vi "PainfulTrial.vi"() -> ()   [LabVIEW 2016]
uses:
  <vilib>/express/express arith-compare/Formula/XNode/ExpressFormulaBlockNode.xnode
panel:
  out "d (m) 2":dbl
  in  "D (in) 2":dbl
  in  "E (psi) 2":dbl
  in  "L (in) 2":dbl
  in  "F (Lbf) 2":dbl
  out "d (m)":dbl
  in  "D (in)":dbl
  in  "E (psi)":dbl
  in  "L (in)":dbl
  in  "F (Lbf)":dbl
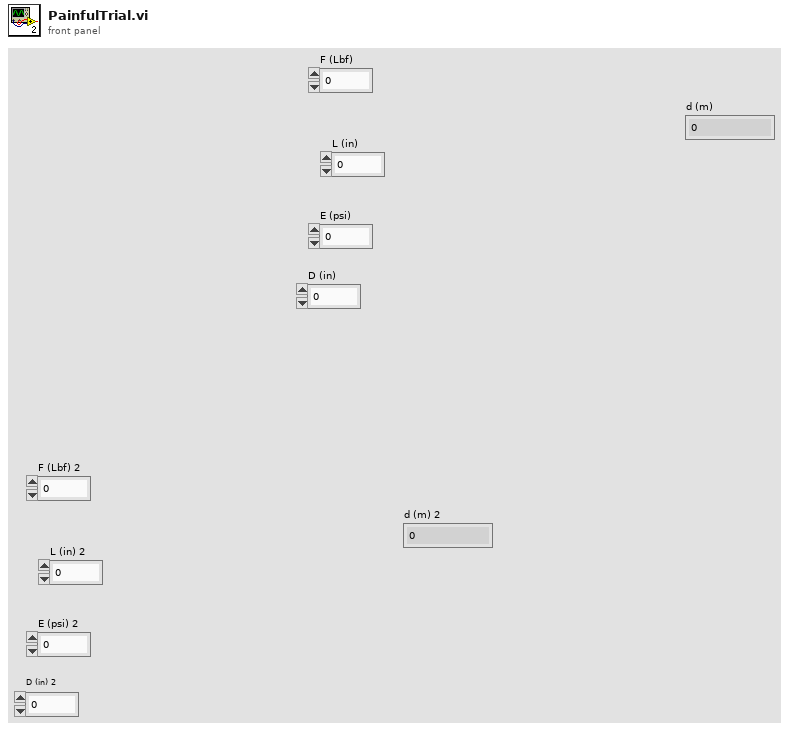
[diagram p1: front panel]
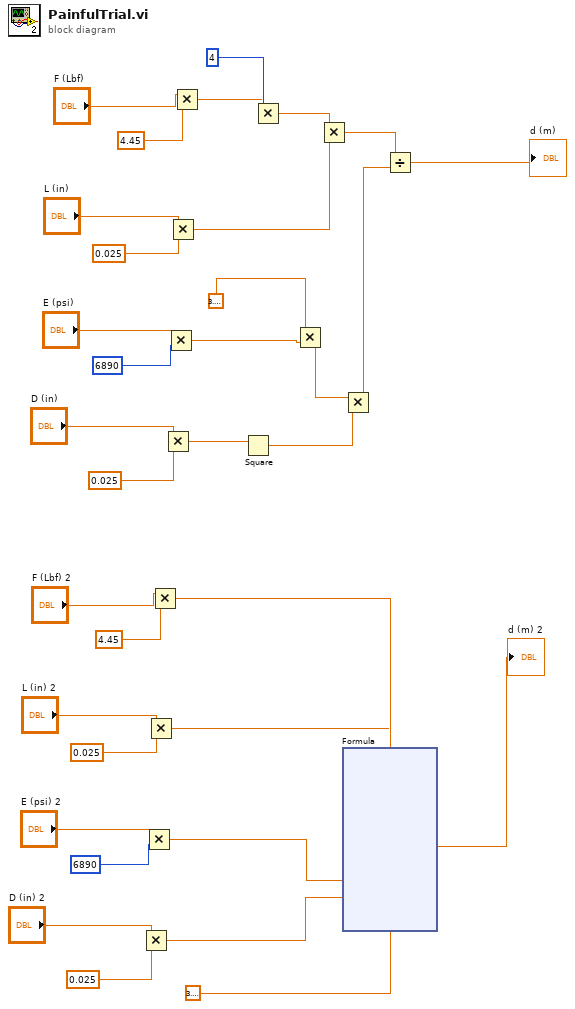
[diagram p0: block diagram]
diagram:
  n1 = Multiply(x="D (in) 2", y=0.025) -> (x*y=w3:dbl)
  n2 = Multiply(x="E (psi) 2", y=6890) -> (x*y=w4:dbl)
  n3 = Multiply(x="L (in) 2", y=0.025) -> (x*y=w5:dbl)
  n4 = Multiply(x="F (Lbf) 2", y=4.45) -> (x*y=w6:dbl)
  n5 = Multiply(x="D (in)", y=0.025) -> (x*y=w21:dbl)
  n6 = Multiply(x="E (psi)", y=6890) -> (x*y=w20:dbl)
  n7 = Multiply(x="L (in)", y=0.025) -> (x*y=w23:dbl)
  n8 = Multiply(x="F (Lbf)", y=4.45) -> (x*y=w25:dbl)
  n9 = Square(x=w21) -> (x^2=w18:dbl)
  n10 = Multiply(x=4, y=w25) -> (x*y=w24:dbl)
  n11 = Multiply(x=3.141592653589793, y=w20) -> (x*y=w19:dbl)
  n12 = Multiply(x=w24, y=w23) -> (x*y=w22:dbl)
  n13 = Multiply(x=w19, y=w18) -> (x*y=w17:dbl)
  n14 = xnode "Formula"("F"=w6, "L"=w5, "E"=w4, "D"=w3, "Pi"=3.141592653589793) -> ("Result"=→"d (m) 2":dbl)  [unwired: 1 in, 1 out]
  n15 = Divide(x=w22, y=w17) -> (x/y=→"d (m)":dbl)
